vi "Encode COB-ID.vi"(9 "Function code":T1=12 items=["EMCY"=1, "PDO1 (tx)"=3, "PDO1 (rx)"=4, "PDO2 (tx)"=5, "PDO2 (rx)"=6, "PDO3 (tx)"=7, "PDO3 (rx)"=8, "PDO4 (tx)"=9, "PDO4 (rx)"=10, "SDO (tx)"=11, "SDO (rx)"=12, "NMT error control"=14], 11 "Node-ID":u8) -> (3 "COD-ID":u32 format="%.0x")   [LabVIEW 2024, in "CANopen Master.lvlib"]
uses:
  CANopen Master.lvlib
  CANopen/FunctionCode.ctl
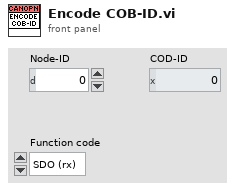
[diagram p1: front panel]
types:
  T1 = typedef "CANopen Master.lvlib/FunctionCode.ctl" = u16
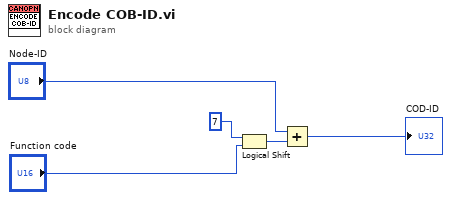
[diagram p0: block diagram]
diagram:
  n1 = Logical Shift(y=i16 7, x="Function code") -> (x << y=w4:T1)
  n2 = Add(x="Node-ID", y=w4) -> (x+y=→"COD-ID":T1)
